vi "Bool to plus minus one.vi"(1 "Boolean":bool) -> (0 "Numeric":dbl)   [LabVIEW 2020]
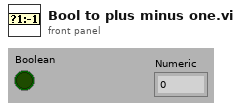
[diagram p1: front panel]
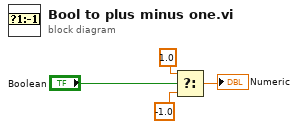
[diagram p0: block diagram]
diagram:
  n1 = Select(t=1.0, s="Boolean", f=-1.0) -> (s? t:f=→"Numeric":dbl)
